vi "init_ccd_sbig.vi"(0 "Scan Directory":string="Peter_ferguson\\Tcal\\scans\\", 1 "Exposure Time":dbl, 2 "Min nm":dbl, 3 "Max nm":dbl, 4 "Step size":dbl, 6 "Scan_prefix":string="test") -> (5 "Working Directory":path)   [LabVIEW 2018]
uses:
  <vilib>/Utility/sysdir.llb/System Directory Type.ctl
panel:
  in  "Name of CCD control code":string="CCDautomation_prefix.exe"
  in  "Boolean":bool=TRUE
  out "Commands Sent":string
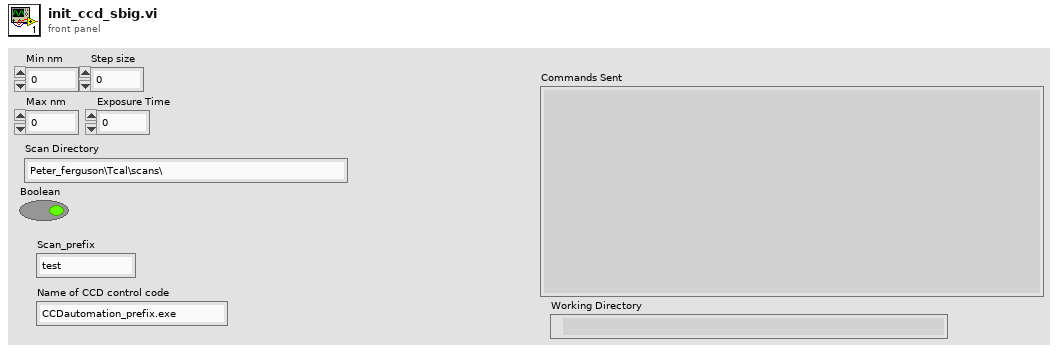
[diagram p1: front panel]
types:
  T1 = enum16{"open", "replace", "create", "open or create", "replace or create", "replace or create with confirmation"}
  T2 = typedef "System Directory Type.ctl" = i32
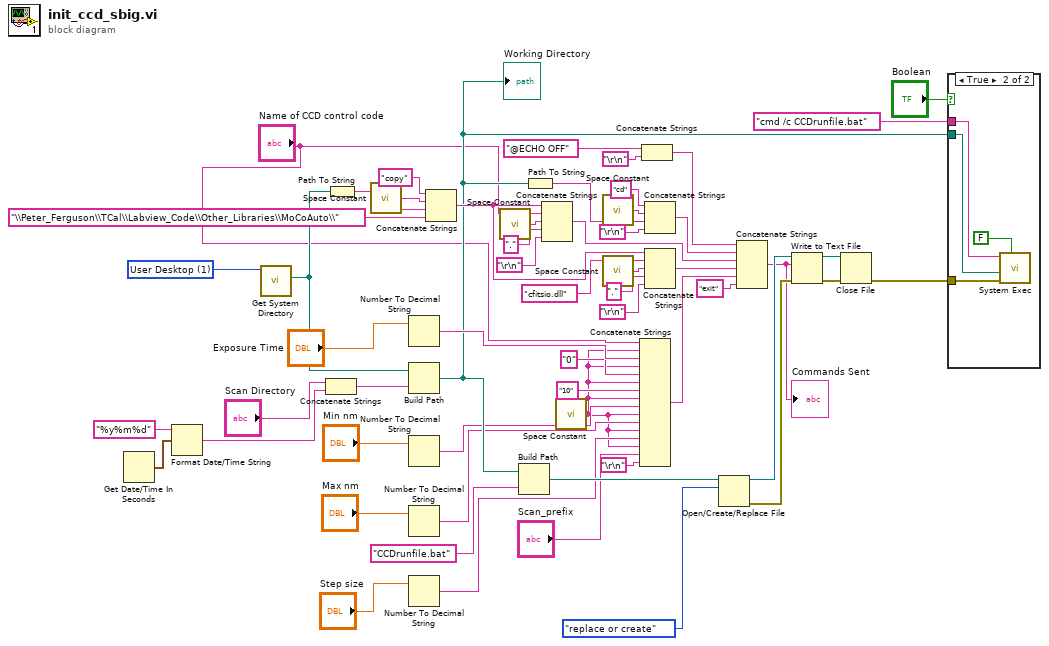
[diagram p0: block diagram]
diagram:
  w55 = T2 1 items=["User Home"=0, "User Desktop"=1, "User Documents"=2, "User Application Data"=3, "User Preferences"=4, "User Temporary"=5, "Public Documents"=6, "Public Application Data"=7, "Public Preferences"=8, "Public Cache"=13, "System Core Libraries"=9, "System Installed Libraries"=10, "Application Files"=11, "Boot Volume Root"=12] ("system directory type")
  n1 = Get Date/Time In Seconds() -> (seconds since 1Jan1904=w57:timestamp)
  n2 = Format Date/Time String(time format string (%c)="%y%m%d", seconds (now)=w57) -> (date/time string=w53:string)  [unwired: 1 in]
  n3 = call <vilib>:"Get System Directory.vi"("system directory type"=w55) -> ("system directory"=w51:path)  [unwired: 10 in]
  n4 = Concatenate Strings("Scan Directory", w53) -> (w52:string)
  n5 = Path To String(path=w51) -> (string=w42:string)
  n6 = call <vilib>:"Space Constant.vi"() -> ("String"=w43:string)
  n7 = Number To Decimal String(number="Exposure Time") -> (decimal integer string=w27:string)  [unwired: 1 in]
  n8 = Build Path(base path=w51, name or relative path=w52) -> (appended path=w14:path)
  "Working Directory" <- w14
  n9 = Number To Decimal String(number="Min nm") -> (decimal integer string=w8:string)  [unwired: 1 in]
  n10 = Number To Decimal String(number="Max nm") -> (decimal integer string=w7:string)  [unwired: 1 in]
  n11 = Number To Decimal String(number="Step size") -> (decimal integer string=w6:string)  [unwired: 1 in]
  n12 = Concatenate Strings("copy", w43, w42, "\\Peter_Ferguson\\TCal\\Labview_Code\\Other_Libraries\\MoCoAuto\\" ("string")) -> (w34:string)
  n13 = call <vilib>:"Space Constant.vi"() -> ("String"=w38:string)
  n14 = Build Path(base path=w14, name or relative path="CCDrunfile.bat") -> (appended path=w21:path)
  n15 = Path To String(path=w14) -> (string=w46:string)
  n16 = Concatenate Strings(w34, "Name of CCD control code", w38, "." ("string"), "\r\n") -> (w35:string)
  n17 = call <vilib>:"Space Constant.vi"() -> ("String"=w4:string)
  n18 = call <vilib>:"Space Constant.vi"() -> ("String"=w47:string)
  n19 = call <vilib>:"Space Constant.vi"() -> ("String"=w32:string)
  n20 = Concatenate Strings("Name of CCD control code", w4, w27, w4, "0" ("string"), w4, "10" ("string"), w4, w8, w4, w7, w4, w6, w4, "Scan_prefix", "\r\n") -> (w11:string)
  n21 = Concatenate Strings("@ECHO OFF" ("string"), "\r\n") -> (w40:string)
  n22 = Concatenate Strings("cd" ("string"), w47, w46, "\r\n") -> (w39:string)
  n23 = Concatenate Strings(w34, "cfitsio.dll" ("string"), w32, "." ("string"), "\r\n") -> (w29:string)
  n24 = Open/Create/Replace File(file path (use dialog)=w21, operation (0:open)=T1."replace or create") -> (refnum out=w18:refnum<file>, error out=w17:errorcluster)  [unwired: 4 in, 1 out]
  n25 = Concatenate Strings(w40, w39, w35, w29, w11, "exit" ("string")) -> (w15:string)
  "Commands Sent" <- w15
  n26 = Write to Text File(file (use dialog)=w18, text=w15, error in=w17) -> (refnum out=w19:refnum<file>, error out=w16:errorcluster)  [unwired: 1 in, 1 out]
  n27 = Close File(refnum=w19, error in=w16) -> (error out=w12:errorcluster)  [unwired: 1 out]
  n28 = case shown="True" "Boolean" {
    tunnel: w14 -> [_ w61]
    tunnel: "cmd /c CCDrunfile.bat" ("command line") -> [_ w60]
    tunnel: w12 -> [_ w58]
    frame False {
    }
    frame True {
      n29 = call <vilib>:"System Exec.vi"("wait until completion? (T)"=FALSE, "error in (no error)"=w58, "working directory"=w61, "command line"=w60) -> ()  [unwired: 4 in, 4 out]
    }
  }
